vi "SVF System Simplified_dynamic.vi"() -> ()   [LabVIEW 2012]
uses:
  <vilib>/addons/Control Design/_Model Construction/Data Typedefs.llb/CD Model Type.ctl
  <vilib>/addons/Control Design/_Model Construction/Model Typedefs.llb/CD Zero-Pole-Gain Model (MIMO).ctl
  <vilib>/addons/Control Design/_Model Construction/Model Typedefs.llb/CD General Elements.ctl
  <vilib>/addons/Control Design/_Model Construction/Model Typedefs.llb/CD Zero-Pole-Gain Model (SISO).ctl
  <vilib>/addons/Control Design/_Model Construction/Model Typedefs.llb/CD State Space Model (MIMO).ctl
  <vilib>/Simulation/Scripting/Companion Diagram/SimConfigNode/SimParams.ctl
  <vilib>/Simulation/Scripting/Companion Diagram/SimConfigNode/_simSolvers.ctl
  <vilib>/Simulation/Implementation/Shared/SIMSCR Execution Mode.ctl
  <vilib>/Simulation/Param Hierarchy/Typedefs/SIMPH Param Control Actions.ctl
  <vilib>/Simulation/Implementation/Shared/NILVSim_ParamChanged.vi
  <vilib>/Simulation/SignalArithmetic/Implementation/NILVSim Gain.llb/SIM Gain (scalar).vi
  <vilib>/Simulation/Utility/Implementation/SIM Halt.vi
  <vilib>/Simulation/DiscreteLinear/Implementation/NILVSim Discrete State Space Buffered.llb/SIM Discrete State Space Distributor (SISO CD).vi
  <vilib>/Simulation/SignalArithmetic/Implementation/NILVSim Gain.llb/SIM Gain (dot product).vi
  <vilib>/Simulation/DiscreteLinear/Implementation/NILVSim Discrete State Space Buffered.llb/SIM Discrete State Space Collector (SISO CD).vi
  <vilib>/Simulation/SignalDisplay/Implementation/NILVSim Time Waveform.llb/SIM Time Waveform (scalar).vi
  <vilib>/Simulation/Implementation/Shared/NILVSim_Manager.vi
  <vilib>/Simulation/Implementation/Shared/NILVSim_FinalizeModel.vi
  <vilib>/addons/Control Design/_Time Response Analysis/Time Response.llb/Time Response subVI/cd_Step Response (State-Space).vi
  <vilib>/addons/Control Design/_Utility/Model Viewer.llb/Model Viewer SubVI/cd_Draw State-Space Equation (SS).vi
  <vilib>/addons/Control Design/_Dynamic Analysis/Dynamic Analysis.llb/Dynamic Analysis subVI/cd_Pole-Zero Map (State-Space).vi
  <vilib>/addons/Control Design/_Model Conversions/Model Type.llb/Model Conversion SubVI/cd_Convert State-Space to Zero-Pole-Gain Model.vi
  <vilib>/addons/Control Design/_Model Construction/Model Information.llb/Model Information SubVIs/cd_Verify If Discrete (State-Space).vi
  <vilib>/addons/Control Design/_Model Construction/Model Information.llb/Model Information SubVIs/cd_Check State Space Model.vi
  <vilib>/addons/Control Design/_Model Construction/Model Information.llb/Model Information SubVIs/cd_Verify Model Type (SS).vi
  <vilib>/addons/Control Design/_Dynamic Analysis/Dynamic Analysis.llb/Dynamic Analysis subVI/cd_Poles (State-Space).vi
  <vilib>/addons/Control Design/_Model Construction/Model Creation.llb/Model Creation SubVI/cd_Create State Space Model.vi
  <vilib>/addons/Control Design/_Model Conversions/Continuous and Discrete.llb/Continuous and Discrete SubVI/cd_Convert Continuous to Discrete (SS).vi
  <vilib>/Simulation/Implementation/Shared/SIM Unbundle Sim Info.vi
  <vilib>/Utility/error.llb/Clear Errors.vi
  <vilib>/Simulation/Implementation/Shared/NILVSim_GetModelError.vi
  <vilib>/Simulation/Implementation/Shared/SIM Bundle Sim Info.vi
  <vilib>/Simulation/Implementation/Shared/SIMSH Read Queue.vi
  <vilib>/Simulation/Implementation/Shared/NILVSim_Initialize.vi
  <vilib>/Simulation/Utility/Implementation/NILVSim Get Time and IsAcceptedStep.vi
  <vilib>/Simulation/Scripting/Companion Diagram/SimConfigNode/SimDog.xnode
  <vilib>/Simulation/Implementation/XNodeFramework/SimXNode/SimX.xnode
  Program Files/National Instruments/LabVIEW 2012/examples/Control and Simulation/Case Studies/Mechatronics/Inverted Pendulum/subVIs/Draw Linear Inverted Pendulum_sim.vi
  <vilib>/addons/Control Design/_Implementation/CD State Feedback Controller.vi
  <vilib>/addons/Control Design/_Implementation/NI_CD_Implementation.lvlib
  <vilib>/addons/Control Design/_Implementation/CD State Feedback Controller (Single Output).vi
  <vilib>/Simulation/ContinuousLinear/Implementation/NILVSim Transfer Function.llb/SIM Transfer Function (SISO).vi
  <vilib>/addons/Control Design/_Model Construction/NI_LinSys_Model Typedefs.lvlib
  <vilib>/Simulation/ContinuousLinear/Implementation/NILVSim State Space.llb/SIM State Space (CD).vi
  <vilib>/Simulation/ContinuousLinear/Implementation/NILVSim Derivative.llb/SIM derivative (scalar).vi
  <vilib>/Simulation/SignalDisplay/Implementation/NILVSim Time Waveform.llb/SIM Time Waveform (vector).vi
  <vilib>/addons/Control Design/_State Feedback Control/NI_CD_State Feedback Control.lvlib
  <vilib>/addons/Control Design/_Model Construction/NI_LinSys_Model Creation.lvlib
  <vilib>/addons/Control Design/_Dynamic Analysis/NI_CD_Dynamic Analysis.lvlib
  <vilib>/addons/Control Design/_Model Conversions/NI_CD_Continuous and Discrete.lvlib
  <vilib>/addons/Control Design/_State-Space Analysis/NI_CD_State-Space Analysis.lvlib
  <vilib>/addons/Control Design/_Model Construction/NI_LinSys_Model Information.lvlib
  <vilib>/addons/Control Design/_Model Conversions/NI_CD_Model Type.lvlib
  <vilib>/Platform/TimedLoop/XDataNode/wakeup.ctl
  <vilib>/Platform/TimedLoop/XDataNode/XDNodeRunTimeDep.lvlib
  <vilib>/Platform/TimedLoop/XDataNode/nitl_modes.ctl
  <vilib>/Platform/TimedLoop/XDataNode/timing_clust.ctl
  <vilib>/Platform/TimedLoop/XDataNode/XDataNode.xnode
  <vilib>/Simulation/Implementation/Shared/NILVSim_FinishedLate.vi
  <vilib>/Simulation/Implementation/Shared/NI_SIM_Implementation.lvlib
  <vilib>/Simulation/ContinuousLinear/Implementation/NILVSim State Space.llb/SIM State Space Distributor (CD).vi
  <vilib>/Simulation/ContinuousLinear/Implementation/NILVSim State Space.llb/SIM State Space Collector (CD).vi
  <vilib>/Simulation/ContinuousLinear/Implementation/NILVSim Transfer Function.llb/SIM Transfer Function Collector (SISO).vi
  <vilib>/Simulation/ContinuousLinear/Implementation/NILVSim Transfer Function.llb/SIM Transfer Function Distributor (SISO).vi
  <vilib>/Simulation/Implementation/Shared/SIM Fire Discrete SubVI.vi
  <vilib>/Simulation/Scripting/Editor Utilities/SIM subVI execution type.ctl
  <vilib>/Simulation/Scripting/Editor Utilities/SIM subVI tag data.ctl
  <vilib>/addons/Control Design/_Utility/NI_CD_Model Viewer.lvlib
  <vilib>/Simulation/DiscreteLinear/Implementation/NILVSim Discrete State Space Buffered.llb/SIM Discrete State Space Buffered (SISO CD).vi
  <vilib>/addons/Control Design/_Time Response Analysis/NI_CD_Time Response.lvlib
  <vilib>/addons/Control Design/_Model Construction/NI_LinSys_Data Typedefs.lvlib
panel:
  out "Step Response Graph":cluster{"time":dbl[], dbl[]}[](graph)
  in  "Select SV Model":bool=TRUE
  out "Discrete State-Space Model":T1={"properties"={"Model name"="System Model", "Input names"=["u0"], "Output names"=["y0"], "Input Delays"=[0.0], "Output Delays"=[0.0], "Sampling Time"=0.1, "Notes"=""}, "A"=[[1.0, 0.09705751225016658, 0.009648384228931255, 0.00032278803187467067], [0.0, 0.9417009350435251, 0.19169345927190307, 0.009648384228931255], [0.0, -0.0009835254055995163, 1.019619556489737, 0.10065366453071445], [0.0, -0.019540617662783182, 0.39303530277273724, 1.019619556489737]], "B"=[[0.0029424877498334255], [0.05829906495647488], [0.000983525405599516], [0.019540617662783182]], "C"=[[0.0, 0.0, 1.0, 0.0]], "D"=[[0.0]], "StateNames"=["x0", "x1", "x2", "x3"], "Transport Delay"=[[0.0]]} {"Transport Delay" format="%.2f"; "D" format="%#.2g"; "C" format="%#.2g"; "B" format="%#.2g"; "A" format="%#.2g"; "properties"."Sampling Time" format="%#.6p"; "properties"."Output Delays" format="%.4f"; "properties"."Input Delays" format="%.4f"}
  in  "Halt?":bool
  out "state x(k)":dbl[](array[numeric])
  out "Discrete Model Out":picture
  in  "Input Signal (IMU)":dbl(slide) scale=-0.1..0.1
  out "Waveform Plot":waveform(dbl)(graph)={"t0"=timestamp(19414.600000000002 s since 1904-01-01), "dt"=1.0, "Y"=[0.0]}
  in  "Inertia of pendulum (I)":dbl=0.8
  in  "Length to center of mass (l)":dbl=0.5
  in  "Kinetic friction of robot (b)":dbl=0.4
  in  "Mass of Rest (m)":dbl=9.0
  in  "Mass of Bottom Wheel (M)":dbl=2.0
  out "Pole-Zero Map":cluster{dbl[], dbl[]}[](graph)=[{[1.2142841528821395, 0.8147971273698099, 0.9518587677710494, 1.0], [0.0, 0.0, 0.0, 0.0]}, {[1.0, 1.0, -0.980160788537376], [0.0, 0.0, 0.0]}]
  out "Zero-Pole-Gain Model":T3={"properties"={"Model name"="System Model", "Input names"=["u0"], "Output names"=["y0"], "Input Delays"=[0.0], "Output Delays"=[0.0], "Sampling Time"=0.1, "Notes"=""}, "zero-pole-gain(s)"=[[{"Gain"=0.000983525405599206, "Zeros"=[0.999999999999886+0.0i, -0.9801607885382041+0.0i], "Poles"=[0.8147971273698099+0.0i, 0.9518587677710494+0.0i, 1.2142841528821395+0.0i], "delay"=0.0}]]} {"zero-pole-gain(s)"."delay" format="%.4f"; "zero-pole-gain(s)"."Poles" format="%#.8g"; "zero-pole-gain(s)"."Zeros" format="%#.8g"; "zero-pole-gain(s)"."Gain" format="%#.8g"; "properties"."Sampling Time" format="%#.6p"; "properties"."Output Delays" format="%.4f"; "properties"."Input Delays" format="%.4f"}
  out "Static Gain Case?":bool
  out "Type of Model":T5=1 items=["Empty", "SISO", "SIMO", "MISO", "MIMO", "Undetermined"]
  out "Number of Outputs":i32=1
  out "Number of Inputs":i32=1
  out "Number of States":i32=4
  out "Sampling Time Required":dbl=0.1 format="%.2f"
  out "Discrete?":bool=TRUE
  out "Controllability Matrix":dbl[][](array[numeric])=[[0.0029424877498334255, 0.008616646869548867, 0.014016016852462686, 0.019193532183387766], [0.05829906495647488, 0.05527735475623796, 0.052797981566245, 0.05083784073300338], [0.000983525405599516, 0.0029123179012991098, 0.004844756877997715, 0.006861898357198368], [0.019540617662783182, 0.019171356382024756, 0.019611979984952656, 0.02086921364939449]] format="%.2f"
  out "Outputs":dbl[](array[numeric])
  out "Plot X and Theta":waveform(dbl)[](graph)=[{"t0"=timestamp(4.71 s since 1904-01-01), "dt"=1.0, "Y"=[-0.13996665083491025]}, {"t0"=timestamp(4.71 s since 1904-01-01), "dt"=1.0, "Y"=[-1.62298383744272e-05]}]
  in  "stop":bool
  in  "Tab Control":T6(tab)=enum."Controller"
  out "System Poles":cdb[](array[numeric])=[1.2142841528821395+0.0i, 0.8147971273698099+0.0i, 0.9518587677710494+0.0i, 1.0+0.0i] format="%#.2g"
  in  "Desired Poles":cdb[](array[numeric])=[-5.0+0.0i, -5.0+0.0i, -20.0+0.0i, -15.0+0.0i] format="%#.2g"
  out "Calculated Poles":cdb[](array[numeric])=[-20.00002973836509+0.0i, -14.99996105048431+0.0i, -5.004299732705596+0.0i, -4.995709482028461+0.0i] format="%#.2g"
  in  "Initial Conditions":T7
  in  "Set Point (m)":dbl(slide)=-0.14 scale=-0.2..0.2
  out "Feedback Gain (K)":dbl[](array[numeric])=[-63312112.22140336, 6720868.965421855, 193328496.30508494, -20246021.6652911]
  out "Boundary Reached":bool
  in  "Discrete Mode":bool=TRUE
  in  "A":dbl[][](array[numeric])=[[0.0, 1.0, 0.0, 0.0], [0.0, -0.1818, 2.6727, 0.0], [0.0, 0.0, 0.0, 1.0], [0.0, -0.4545, 31.1818, 0.0]] format="%#.2g"
  in  "B":dbl[][](array[numeric])=[[0.0], [1.8182], [0.0], [4.5455]] format="%#.2g"
  in  "C":dbl[][](array[numeric])=[[1.0, 0.0, 0.0, 0.0], [0.0, 0.0, 1.0, 0.0]] format="%#.2g"
  in  "D":dbl[][](array[numeric])=[[0.0], [0.0]] format="%#.2g"
  in  "Sampling Time (s)":dbl=0.1
  out "3D Picture Control":refnum<vi>(3d-picture)
  # "MODEL INFO"
  # "DISCRETE INFO"
  # "If you installed the LabVIEW Control Design Toolkit, you can design a controller by specifying the locations of the Desired Poles.\n\nOtherwise, click the Controller tab to specify the controller Feedback Gain."
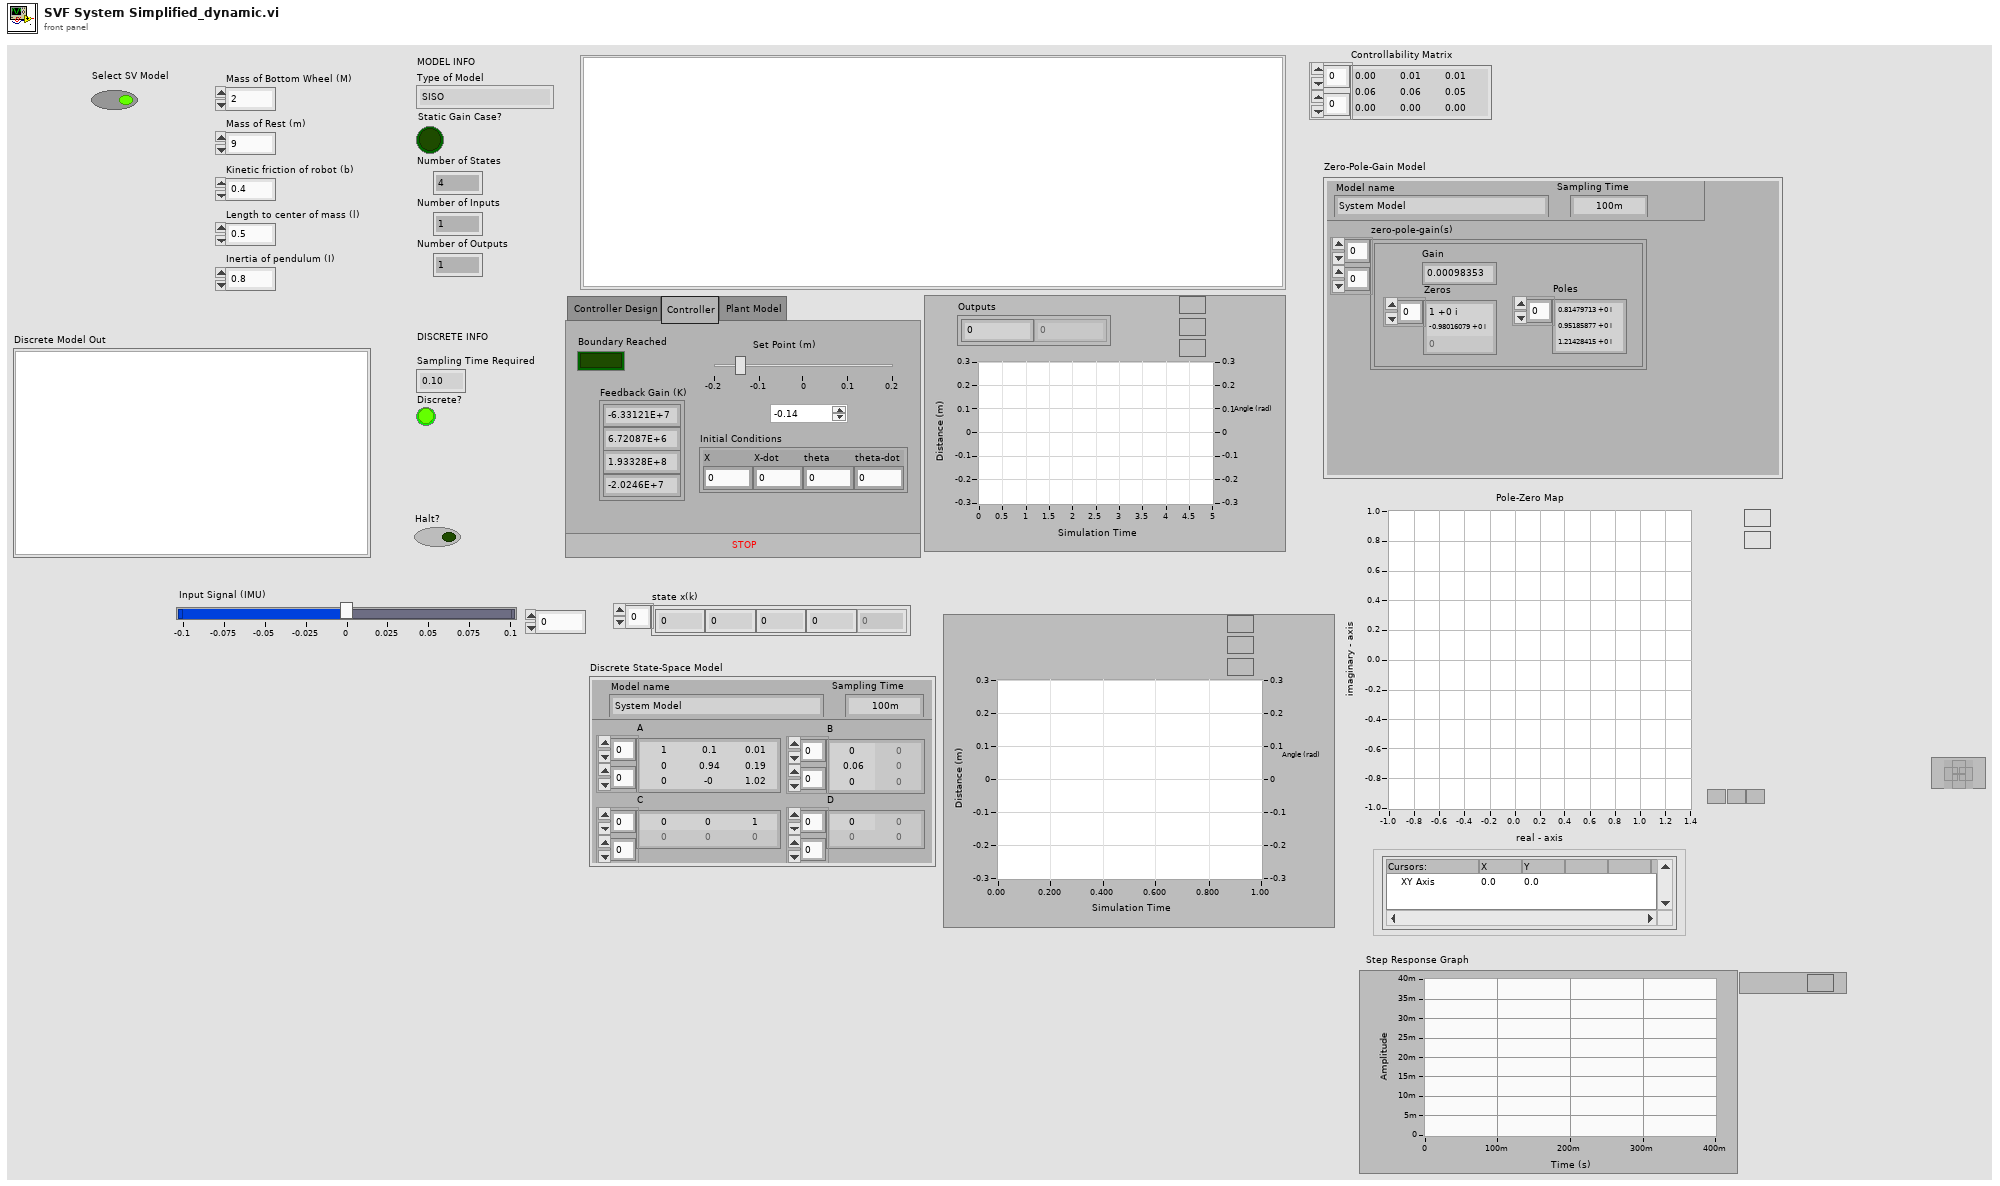
[diagram p1: front panel]
types:
  T1 = typedef "NI_LinSys_Model Typedefs.lvlib/CD State Space Model (MIMO).ctl" = cluster{"properties":T2, "A":dbl[][], "B":dbl[][], "C":dbl[][], "D":dbl[][], "StateNames":string[], "Transport Delay":dbl[][]}
  T2 = typedef "NI_LinSys_Model Typedefs.lvlib/CD General Elements.ctl" = cluster{"Model name":string, "Input names":string[], "Output names":string[], "Input Delays":dbl[], "Output Delays":dbl[], "Sampling Time":dbl, "Notes":string}
  T3 = typedef "NI_LinSys_Model Typedefs.lvlib/CD Zero-Pole-Gain Model (MIMO).ctl" = cluster{"properties":T2, "zero-pole-gain(s)":T4[][]}
  T4 = typedef "NI_LinSys_Model Typedefs.lvlib/CD Zero-Pole-Gain Model (SISO).ctl" = cluster{"Gain":dbl, "Zeros":cdb[], "Poles":cdb[], "delay":dbl}
  T5 = typedef "NI_LinSys_Data Typedefs.lvlib/CD Model Type.ctl" = u16
  T6 = enum32{"Controller Design", "Controller", "Plant Model"}
  T7 = cluster{"X":dbl, "X-dot":dbl, "theta":dbl, "theta-dot":dbl}
  T8 = typedef "SIMSCR Execution Mode.ctl" = enum16{"Simulate to Completion", "Single Time-Step Simulation (Fixed Step Only)"}
  T9 = typedef "XDNodeRunTimeDep.lvlib/timing_clust.ctl" = cluster{"Expected End [f-1]":u64, "Actual End [f-1]":u64, "Finished Late? [f-1]":bool, "Expected End [i-1]":u64, "Actual End [i-1]":u64, "Finished Late? [i-1]":bool, "Expected Start [i]":u64, "Actual Start [i]":u64, "Expected Start [f]":u64, "Actual Start [f]":u64, "Source Name":string, "Structure Name":string, "Period":i64, "Deadline":i64, "Offset":i64, "Start":i64, "Priority":i32, "Timeout":i32, "Mode":T10, "Wakeup Reason":T11, "Error":errorcluster, "Source Type":string, "Secondary Source Type":string, "Global End Time":u64, "Global Start Time":u64, "Frame Duration":u64, "Iteration Duration":u64, "Assigned CPU":i32, "I/O Scan Engine Mode":u32}
  T10 = typedef "XDNodeRunTimeDep.lvlib/nitl_modes.ctl" = enum32{"No Change", "Process missed periods, maintain original phase", "Discard missed periods, maintain original phase", "Process missed periods, ignore original phase", "Discard missed periods, ignore original phase"}
  T11 = typedef "XDNodeRunTimeDep.lvlib/wakeup.ctl" = enum32{"Normal", "Aborted", "Asynchronous wakeup", "Timing source error", "Timed loop error", "Timeout"}
  T12 = typedef "SIMPH Param Control Actions.ctl" = enum16{"get params", "set params"}
  T13 = typedef "SIM subVI tag data.ctl" = cluster{"period":dbl, "skew":dbl, "Simulation execution type":T14}
  T14 = typedef "SIM subVI execution type.ctl" = enum16{"Function call", "Discrete", "Continuous", "Initialization only", "Final step only"}
  T15 = typedef "SimParams.ctl" = cluster{"Initial Time (s)":dbl, "Final Time (s)":dbl, "Step Size (s)":dbl, "ODE Solver":T16, "Minimum Step Size (s)":dbl, "Maximum Step Size (s)":dbl, "Relative Tolerance":dbl, "Absolute Tolerance":dbl, "Software Timing":bool, "Initial Step Size (s)":dbl, "Automatic Fixed Step Size?":bool, "Automatic Discrete Step Size?":bool, "Discrete Step Size (s)":dbl, "Calculate using Time Step":bool, "Solver Wired?":bool, "Prev.Frm.Expected End":u64, "Prev.Frm.Actual End":u64, "Prev.Frm.Finished Late?":bool, "Prev.Iter.Expected End":u64, "Prev.Iter.Actual End":u64, "Prev.Iter.Finished Late?":bool, "Expected Iteration Start":u64, "Actual Iteration Start":u64, "Expected Frame Start":u64, "Actual Frame Start":u64, "Source Name":string, "Name":string, "Period":i64, "Deadline":i64, "Offset":i64, "Start":i64, "Priority":i32, "Timeout":i32, "Processor":i32, "Mode":enum32{"No Change", "Process missed periods, maintain original phase", "Discard missed periods, maintain original phase", "Process missed periods, ignore original phase", "Discard missed periods, ignore original phase"}, "Wakeup reason":enum32{"Normal", "Aborted", "Asynchronous wakeup", "Timing source error", "Timed loop error", "Timeout"}, "Error":errorcluster, "Source Type":string, "Secondary Source Type":string, "Global End Time":u64, "Global Start Time":u64, "Full Solver Reset":bool, "Execution Mode":T8, "Nan/Inf Check":bool, "Custom Solver Library":string, "Solver Is Variable":bool, "custom solver name":string, "Signal Collection Decimation":u32}
  T16 = typedef "_simSolvers.ctl" = enum16{"Runge-Kutta 1 (Euler)", "Runge-Kutta 2", "Runge-Kutta 3", "Runge-Kutta 4", "Runge-Kutta 23 (variable)", "Runge-Kutta 45 (variable)", "BDF (variable)", "Adams-Moulton (variable)", "Rosenbrock (variable)", "Discrete States Only", "SDIRK 4 (variable)", "Radau 5 (variable)", "Radau 9 (variable)", "Radau 13 (variable)", "Radau [Variable Order] (variable)", "Gear's Method (variable)", "Linearizer", "State Query", "Trim Eval", "Custom Solver"}
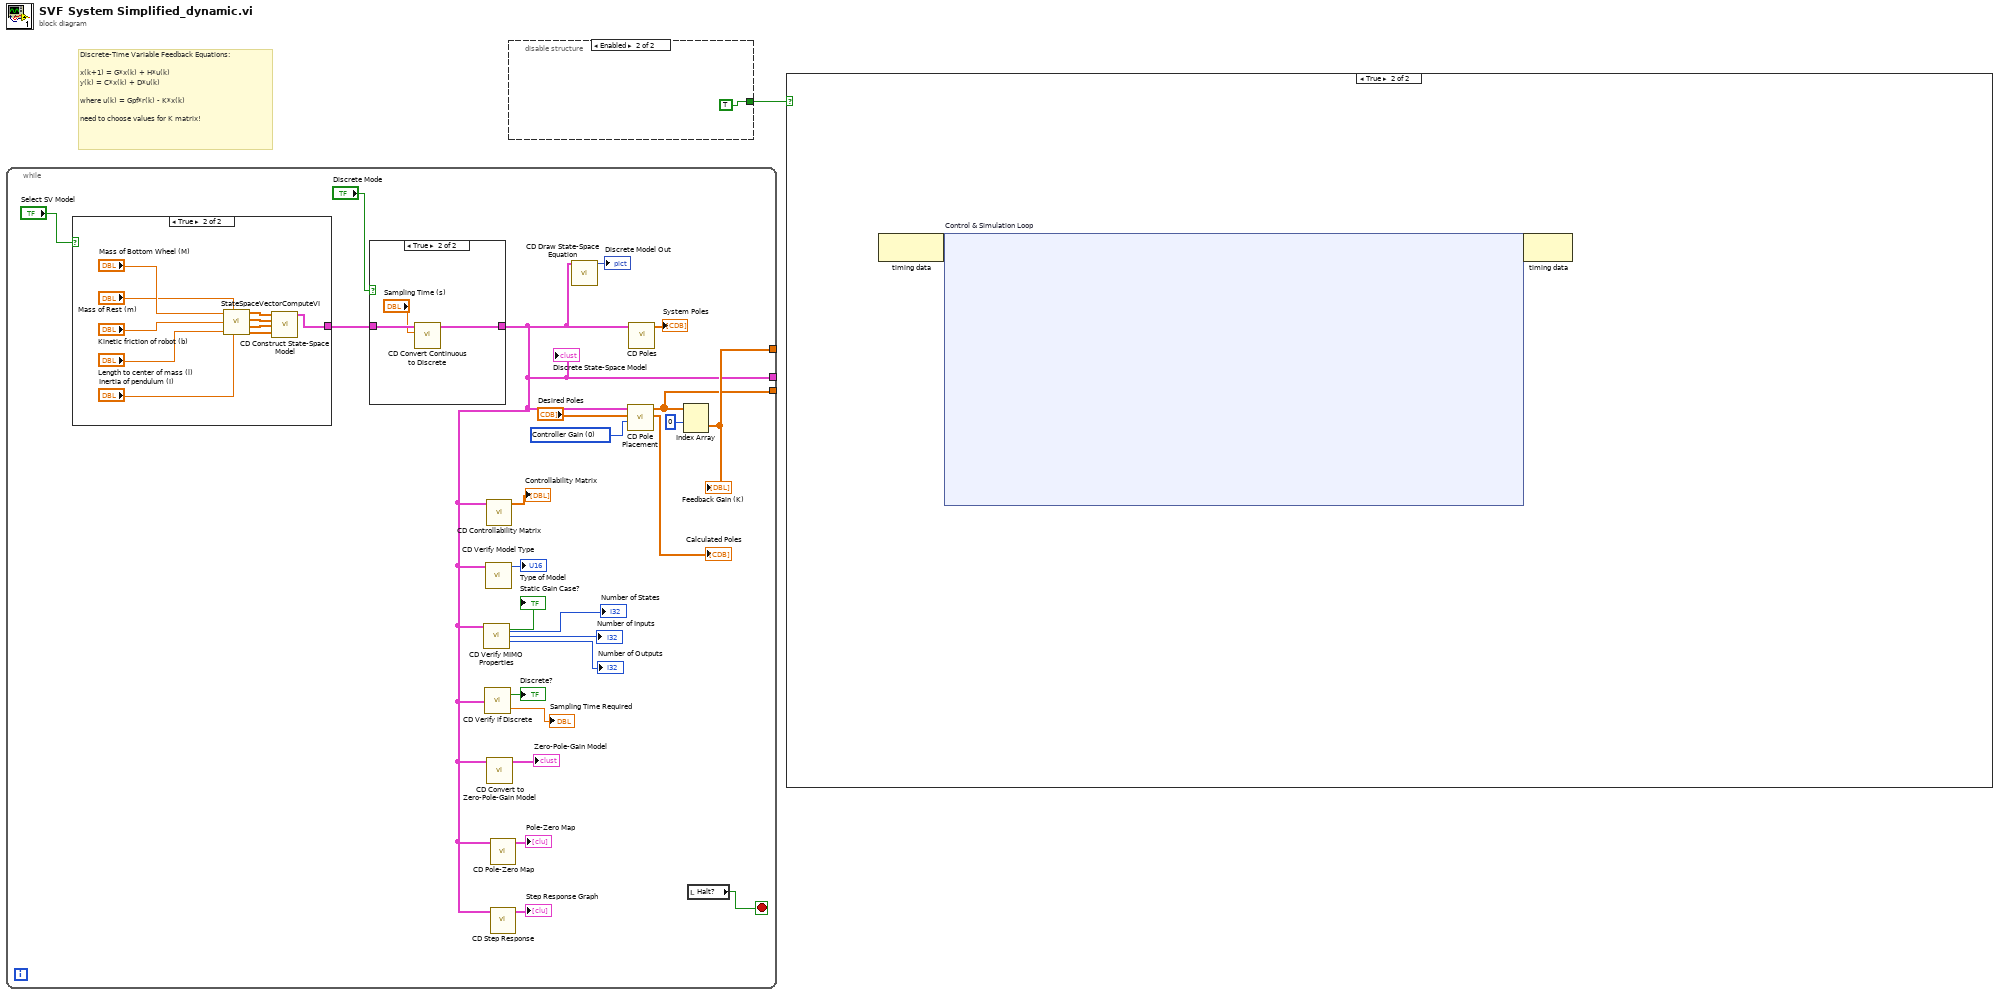
[diagram p0: block diagram]
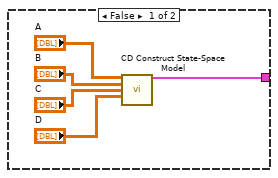
[diagram p2: hidden frame]
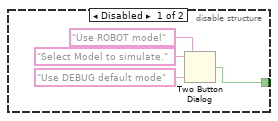
[diagram p4: hidden frame]
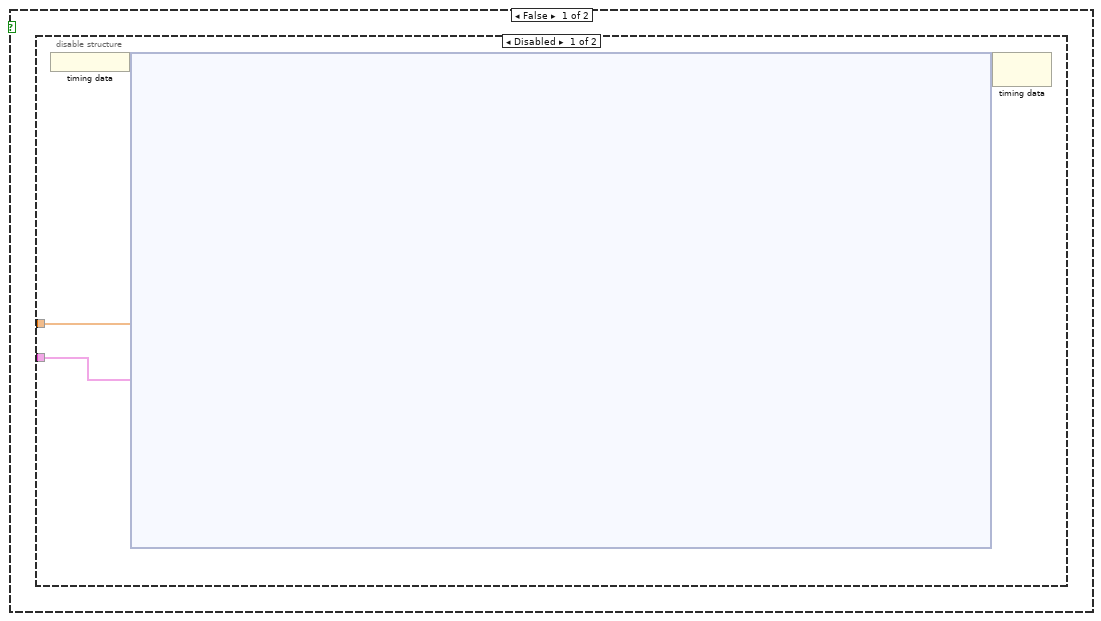
[diagram p5: hidden frame]
diagram:
  # "Discrete-Time Variable Feedback Equations:\n\nx(k+1) = G*x(k) + H*u(k)\ny(k) = C*x(k) + D*u(k)\n\nwhere u(k) = Gpf*r(k) - K*x(k)\n\nneed to choose values for K matrix!"
  n1 = while {
    tunnel: [w20] -> _
    tunnel: [w7] -> _
    tunnel: [w3] -> _
    stop <- w5 stop-if-true
    w25 = u16 0 items=["Controller Gain", "Observer Gain (Predictive)", "Observer Gain (Current)"] ("Gain Type")
    n2 = case shown="True" "Select SV Model" {
      tunnel: [w26 w31] -> w19
      frame False {
        n3 = call-poly <vilib>:"CD Construct State-Space Model.vi"("A"="A", "B"="B", "C"="C", "D"="D") -> ("State-Space Model"=w26:T1)  [unwired: 10 in, 1 out]
      }
      frame True {
        n4 = call "StateSpaceVectorComputeVI.vi"("Mass of Bottom Wheel (M)"="Mass of Bottom Wheel (M)", "Mass of Rest (m)"="Mass of Rest (m)", "Kinetic friction of robot (b)"="Kinetic friction of robot (b)", "Length to center of mass (l)"="Length to center of mass (l)", "Inertia of pendulum (I)"="Inertia of pendulum (I)") -> ("A"=w35:dbl[][], "B"=w34:dbl[][], "C"=w33:dbl[][], "D"=w32:dbl[][])
        n5 = call-poly <vilib>:"CD Construct State-Space Model.vi"("A"=w35, "B"=w34, "C"=w33, "D"=w32) -> ("State-Space Model"=w31:T1)  [unwired: 10 in, 1 out]
      }
    }
    n6 = case shown="True" "Discrete Mode" {
      tunnel: w19 -> [w41 w44]
      tunnel: [w41 w42] -> w3
      frame False {
      }
      frame True {
        n7 = call-poly <vilib>:"CD Convert Continuous to Discrete.vi"("Sampling Time (s)"="Sampling Time (s)", "Continuous State-Space Model"=w44) -> ("Discrete State-Space Model"=w42:T1)  [unwired: 7 in, 2 out]
      }
    }
    "Discrete State-Space Model" <- w3
    n8 = call-poly <vilib>:"CD Verify MIMO Properties.vi"("State-Space Model In"=w3) -> ("Static Gain Case?"=→"Static Gain Case?":bool, "Number of States"=→"Number of States":i32, "Number of Inputs"=→"Number of Inputs":i32, "Number of Outputs"=→"Number of Outputs":i32)  [unwired: 9 in, 2 out]
    n9 = call-poly <vilib>:"CD Verify if Discrete.vi"("State-Space Model"=w3) -> ("Discrete?"=→"Discrete?":bool, "Sampling Time"=→"Sampling Time Required":dbl)
    n10 = call-poly <vilib>:"CD Verify Model Type.vi"("State-Space Model"=w3) -> ("Type of Model"=→"Type of Model":T5)  [unwired: 9 in, 1 out]
    n11 = call <vilib>:"CD Controllability Matrix.vi"("State-Space Model"=w3) -> ("Controllability Matrix"=→"Controllability Matrix":dbl[][])  [unwired: 7 in, 3 out]
    n12 = call-poly <vilib>:"CD Convert to Zero-Pole-Gain Model.vi"("State-Space Model"=w3) -> ("Zero-Pole-Gain Model"=→"Zero-Pole-Gain Model":T3)  [unwired: 9 in, 1 out]
    n13 = call-poly <vilib>:"CD Pole-Zero Map.vi"("State-Space Model"=w3) -> ("Pole-Zero Map"=→"Pole-Zero Map":cluster{dbl[], dbl[]}[])  [unwired: 7 in, 3 out]
    n14 = call-poly <vilib>:"CD Step Response.vi"("State-Space Model"=w3) -> ("Step Response Graph"=→"Step Response Graph":cluster{"time":dbl[], dbl[]}[])  [unwired: 7 in, 3 out]
    n15 = call-poly <vilib>:"CD Draw State-Space Equation.vi"("State-Space Model"=w3) -> ("Equation"=→"Discrete Model Out":picture)  [unwired: 8 in, 2 out]
    n16 = call <vilib>:"CD Pole Placement.vi"("Gain Type"=w25, "Poles"="Desired Poles", "State-Space Model"=w3) -> ("Actual Poles"=→"Calculated Poles":cdb[], "Gain"=w7:dbl[][])  [unwired: 6 in, 1 out]
    n17 = call-poly <vilib>:"CD Poles.vi"("State-Space Model"=w3) -> ("Poles"=→"System Poles":cdb[])  [unwired: 9 in, 1 out]
    n18 = Index Array(array=w7, index (row)=0) -> (element=w20:dbl[])  [unwired: 1 in]
    "Feedback Gain (K)" <- w20
    n19 = local read "Halt?"() -> (w5:bool)
  }
  n20 = disable-structure shown="Enabled" {
    disable-tunnel: [w48 TRUE ("T button?")] -> w1
    frame Disabled {
      n21 = Two Button Dialog(message="Select Model to simulate.", 1:"Use DEBUG default mode" ("F button name (\"Cancel\")"), 2:"Use ROBOT model" ("T button name (\"OK\")")) -> (T button?=w48:bool)
    }
    frame Enabled {
    }
  }
  n22 = case shown="True" w1 {
    frame False {
      n23 = disable-structure shown="Disabled" {
        disable-tunnel: _ -> [w51 _]
        disable-tunnel: _ -> [w50 _]
        frame Disabled {
          n24 = node-c288() -> (w53:variant)
          n25 = node-c254 ("Simulation Loop")(w53, w50, w51) -> (w52:variant)
          n26 = node-c288(w52) -> ()  [unwired: 1 out]
        }
        frame Enabled {
        }
      }
    }
    frame True {
      n27 = node-c288() -> (w455:variant)  [unwired: 1 in]
      n28 = node-c254 "Control & Simulation Loop"(w455) -> (w454:variant)
      n29 = node-c288(w454) -> ()  [unwired: 1 out]
    }
  }
